vi "DLOD Cards.vi"() -> ()   [LabVIEW 2024]
doc: "Demonstrates the usage of \"IMAQ DL Model Detect Objects\" to perform Object Detection using Deep Learning for Defect Inspection application."
uses:
  <vilib>/userDefined/High Color/IMAQdx.ctl
  <vilib>/Python/Open Anaconda Python Session.vi
  <vilib>/vision/driver/NI_Vision_Acquisition_Software.lvlib
  <vilib>/vision/NI_Vision_Development_Module.lvlib
panel:
  in  "Model Path":path=path "C:/Users/cesar/Final/cards_model"
  out "Iteraciones":i32
  in  "Upload":bool
  in  "Card Path":path=path "C:/Users/cesar/Final/reading_card/card.png"
  out "Carta":string
  in  "Anaconda Path":path=path "C:/ProgramData/anaconda3"
  in  "Script Path":path=path "C:/Users/cesar/Final/script_labview.py"
  out "ROI":T1
  in  "Refresh ROI":bool
  out "Image":T2(plugin-control)
  out "error out":errorcluster
  in  "error in":errorcluster
  in  "Stop":bool
  in  "Session":T3="cam0"
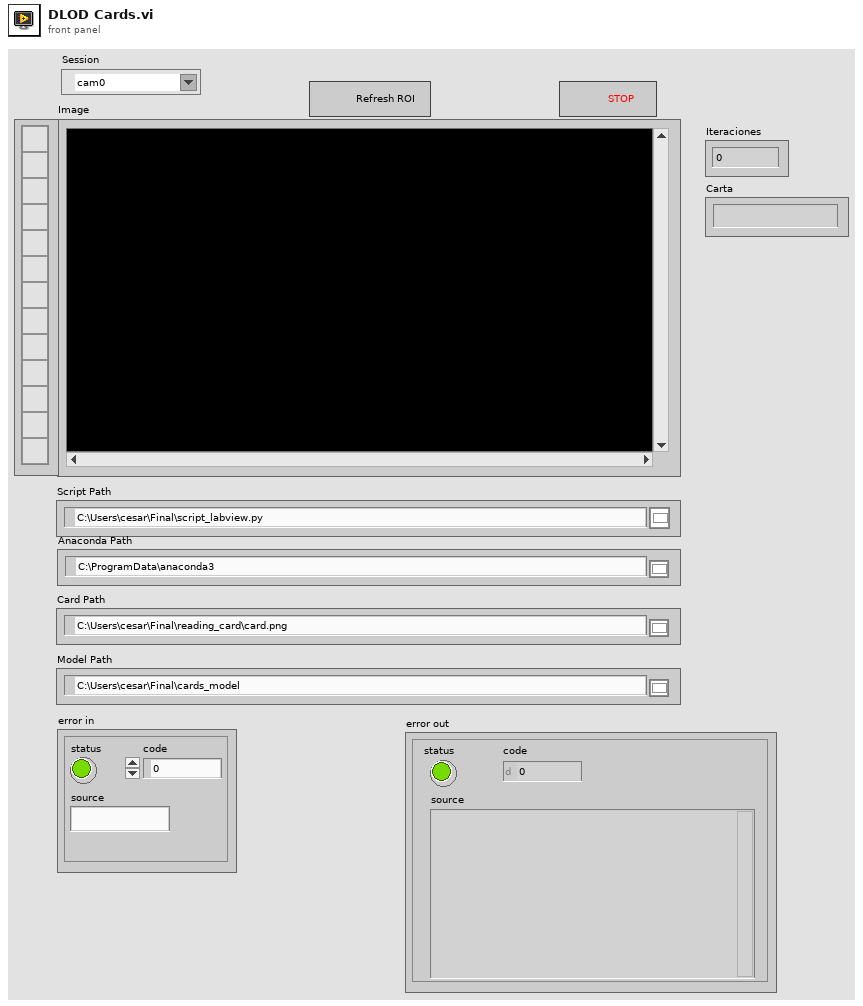
[diagram p1: front panel]
types:
  T1 = cluster{"Global Rectangle":i32[], "Contours":cluster{"Contour Type":u32, "ROI Type":u32, "Points":i32[]}[]}
  T2 = typedef "IMAQ Image.ctl" = refnum<image>
  T3 = typedef "IMAQdx.ctl" = refnum<k21>
  T4 = cluster{"Contour Type":u32, "ROI Type":u32, "Points":i32[]}[]
  T5 = cluster{"Contour Type":u32, "ROI Type":u32, "Points":i32[]}
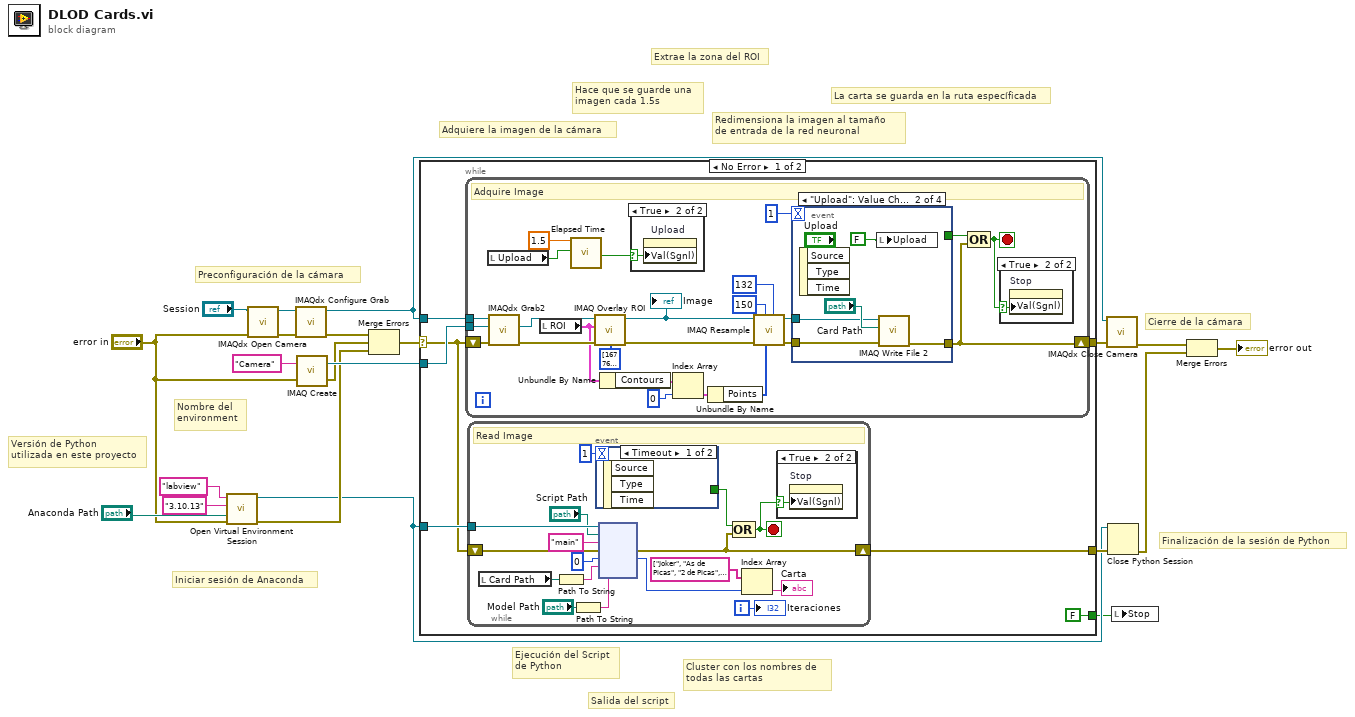
[diagram p0: block diagram]
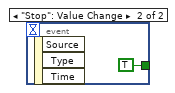
[diagram p3: hidden frame]
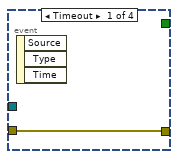
[diagram p6: hidden frame]
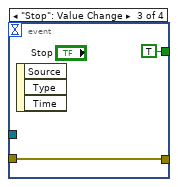
[diagram p7: hidden frame]
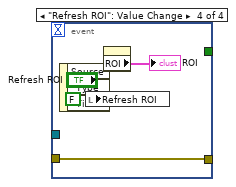
[diagram p8: hidden frame]
diagram:
  # "Salida del script"
  # "Cierre de la cámara"
  # "Finalización de la sesión de Python"
  # "Cluster con los nombres de\ntodas las cartas"
  # "Ejecución del Script\nde Python"
  # "Nombre del\nenvironment"
  # "Versión de Python\nutilizada en este proyecto"
  # "Iniciar sesión de Anaconda"
  # "Preconfiguración de la cámara"
  # "Hace que se guarde una\nimagen cada 1.5s"
  # "La carta se guarda en la ruta específicada"
  # "Redimensiona la imagen al tamaño \nde entrada de la red neuronal"
  # "Extrae la zona del ROI"
  # "Adquiere la imagen de la cámara"
  n1 = call-poly <vilib>:"Open Virtual Environment Session.vi"("error in (no error)"="error in", "Anaconda path"="Anaconda Path", "Python version"="3.10.13", "Env name"="labview") -> ("error out"=w8:errorcluster, "session out"=w3:refnum<k35>)  [unwired: 6 in]
  n2 = call <vilib>:"IMAQdx Open Camera.vi"("error in"="error in", "Session In"="Session") -> ("error out"=w19:errorcluster, "Session Out"=w20:T3)  [unwired: 8 in]
  n3 = call <vilib>:"IMAQdx Configure Grab.vi"("error in"=w19, "Session In"=w20) -> ("error out"=w12:errorcluster, "Session Out"=w14:T3)  [unwired: 8 in]
  n4 = call "IMAQ Create"("Image Name"="Camera", "error in (no error)"="error in") -> ("New Image"=w17:T2, "error out"=w11:errorcluster)  [unwired: 3 in]
  n5 = Merge Errors(w12, w11, w8) -> (w13:errorcluster)
  n6 = case shown="No Error" w13 {
    selector: w13 -> [w24 w85]
    tunnel: w14 -> [w28 _]
    tunnel: w17 -> [w27 _]
    tunnel: [w26 w85] -> w9
    tunnel: w3 -> [w25 _]
    tunnel: [w23 w85] -> w7
    tunnel: [FALSE ("Stop") _] -> w2
    frame No Error {
      n7 = while {
        tunnel: w28 -> [w71]
        shift-right: [w49] -> w26
        shift-left: w24 -> [w70]
        tunnel: w27 -> [w60]
        stop <- w48 stop-if-true
        # "Adquire Image"
        n8 = local read "Upload"() -> (w51:bool)
        n9 = call <vilib>:"IMAQdx Grab2.vi"("error in"=w70, "Image In"=w60, "Session In"=w71) -> ("error out"=w62:errorcluster, "Image Out"=w63:T2)  [unwired: 5 in, 2 out]
        n10 = local read "ROI"() -> (w56:T1)
        n11 = call "Elapsed Time"("Time Target (s)"=1.5, "Reset"=w51) -> ("Time has Elapsed"=w53:bool)  [unwired: 10 in, 7 out]
        n12 = call "IMAQ Overlay ROI"("Colors (Green)"=u32[] [16776002], "error in (no error)"=w62, "ROI Descriptor"=w56, "Image"=w63) -> ("error out"=w59:errorcluster, "Image Out"=w58:T2)  [unwired: 6 in]
        "Image" <- w58
        n13 = Unbundle By Name(w56) -> ("Contours"=w68:T4)
        n14 = case shown="True" w53 {
          selector: w53 -> [_ w73]
          frame False {
          }
          frame True {
            n15 = property on="Upload" class="Bool (strict)"("Val(Sgnl)"=w73) -> ()  [unwired: 2 in, 2 out]
          }
        }
        n16 = Index Array(array=w68, index=0) -> (element=w66:T5)
        n17 = Unbundle By Name(w66) -> ("Points"=w57:i32[])
        n18 = call "IMAQ Resample"("X Resolution"=132 ("X"), "Optional Rectangle"=w57, "Y Resolution"=150 ("Y"), "error in (no error)"=w59, "Image Src"=w58) -> ("error out"=w54:errorcluster, "Image Dst Out"=w55:T2)  [unwired: 5 in]
        n19 = event shown="[1] \"Upload\": Value Change" {
          selector: _ -> [_ _ _ _]
          dyn-events: _ -> [_ _ _ _]
          timeout: 1 -> [_ _ _ _]
          tunnel: [_ _ TRUE ("Stop") _] -> w50
          tunnel: w55 -> [_ w77 _ _]
          tunnel: w54 -> [w74 w76 w80 w82]
          tunnel: [w74 w75 w80 w82] -> w49
          event Timeout {
            n20 = event-data() -> ()  [unwired: 1 in, 3 out]
          }
          event "Upload": Value Change {
            n21 = event-data() -> ()  [unwired: 1 in, 3 out]
            n22 = local write "Upload"(FALSE ("Upload")) -> ()
            n23 = call-poly "IMAQ Write File 2"("error in (no error)"=w76, "File Path"="Card Path", "Image"=w77) -> ("error out"=w75:errorcluster)  [unwired: 7 in, 1 out]
          }
          event "Stop": Value Change {
            n24 = event-data() -> ()  [unwired: 1 in, 3 out]
          }
          event "Refresh ROI": Value Change {
            n25 = event-data() -> ()  [unwired: 1 in, 3 out]
            n26 = local write "Refresh ROI"(FALSE ("Refresh ROI")) -> ()
            n27 = property on="Image" class="ImageControl"() -> ("ROI"=→"ROI":T1)  [unwired: 2 in, 2 out]
          }
        }
        n28 = Compound Arithmetic op=OR(w50, w49) -> (w48:bool)
        n29 = case shown="True" w48 {
          selector: w48 -> [_ w72]
          frame False {
          }
          frame True {
            n30 = property on="Stop" class="Bool (strict)"("Val(Sgnl)"=w72) -> ()  [unwired: 2 in, 2 out]
          }
        }
      }
      n31 = while {
        tunnel: w25 -> [w40]
        shift-right: [w37] -> w23
        shift-left: w24 -> [w38]
        i -> [w34]
        stop <- w31 stop-if-true
        # "Read Image"
        n32 = local read "Card Path"() -> (w36:path)
        n33 = Path To String(path=w36) -> (string=w35:string)
        n34 = Path To String(path="Model Path") -> (string=w30:string)
        n35 = event shown="[0] Timeout" {
          selector: _ -> [_ _]
          dyn-events: _ -> [_ _]
          timeout: 1 -> [_ _]
          tunnel: [_ TRUE] -> w32
          event Timeout {
            n36 = event-data() -> ()  [unwired: 1 in, 3 out]
          }
          event "Stop": Value Change {
            n37 = event-data() -> ()  [unwired: 1 in, 3 out]
          }
        }
        n38 = node(w40, "Script Path", "main" ("function name"), w38, 0 ("Salida"), w35, w30) -> (w37:errorcluster, w44:i32)  [unwired: 2 in, 3 out]
        n39 = Compound Arithmetic op=OR(w32, w37) -> (w31:bool)
        n40 = Index Array(array=string[] ["Joker", "As de Picas", "2 de Picas", "3 de Picas", "4 de Picas", "5 de Picas", "6 de Picas", "7 de Picas", "8 de Picas", "9 de Picas", "10 de Picas", "J de Picas", "Q de Picas", "K de Picas", "As de Corazones", "2 de Corazones", "3 de Corazones", "4 de Corazones", "5 de Corazones", "6 de Corazones", "7 de Corazones", "8 de Corazones", "9 de Corazones", "10 de Corazones", "J de Corazones", "Q de Corazones", "K de Corazones", "As de Tréboles", "2 de Tréboles", "3 de Tréboles", "4 de Tréboles", "5 de Tréboles", "6 de Tréboles", "7 de Tréboles", "8 de Tréboles", "9 de Tréboles", "10 de Tréboles", "J de Tréboles", "Q de Tréboles", "K de Tréboles", "As de Diamantes", "2 de Diamantes", "3 de Diamantes", "4 de Diamantes", "5 de Diamantes", "6 de Diamantes", "7 de Diamantes", "8 de Diamantes", "9 de Diamantes", "10 de Diamantes", "J de Diamantes", "Q de Diamantes", "K de Diamantes"], index=w44) -> (element=→"Carta":string)
        n41 = case shown="True" w31 {
          selector: w31 -> [_ w46]
          frame False {
          }
          frame True {
            n42 = property on="Stop" class="Bool (strict)"("Val(Sgnl)"=w46) -> ()  [unwired: 2 in, 2 out]
          }
        }
        "Iteraciones" <- w34
      }
    }
    frame Error {
      n43 = call <vilib>:"Simple Error Handler.vi"("error in (no error)"=w85) -> ()  [unwired: 4 in, 5 out]
    }
  }
  n44 = call <vilib>:"IMAQdx Close Camera.vi"("error in"=w9, "Session In"=w14) -> ("error out"=w6:errorcluster)  [unwired: 9 in]
  n45 = Close Python Session(session in=w3, error in=w7) -> (11:w4:errorcluster)
  n46 = local write "Stop"(w2) -> ()
  n47 = Merge Errors(w6, w4) -> (→"error out":errorcluster)
